vi "Patch data preview-Initialise all.vi"() -> (2 "VL array refs":T1[](array[typedef]), 3 "U8 Image ref":T1)   [LabVIEW 2020]
uses:
  <vilib>/vision/Image Controls.llb/IMAQ Image.ctl
  User Interface/Visualisation/Timelapse Viewer/Globals/gl_Time series viewer globals.vi
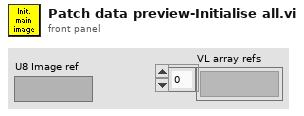
[diagram p1: front panel]
types:
  T1 = typedef "IMAQ Image.ctl" = refnum<image>
  T2 = typedef "Time series viewer refs.ctl" = cluster{"This VI":refnum<vi>, "Image control":refnum<vi>, "AVI Mode ind":refnum<vi>, "Play":refnum<vi>, "Stop":refnum<vi>, "Back":refnum<vi>, "Scrollbar":refnum<vi>, "Video length info":refnum<vi>, "Expected speed values":refnum<vi>, "Intensity":refnum<vi>, "Path":refnum<vi>, "Selection sliders":refnum<vi>, "Speed Graph ref":refnum<vi>, "Frame rate set (fps)":refnum<vi>, "Number of rows to generate":refnum<vi>, "VL Image Array":refnum<vi>, "Image Scrollbar":refnum<vi>, "Channel to load":refnum<vi>, "Colour":refnum<vi>}
  T3 = typedef "Channel to load.ctl" = enum16{"Show red channel", "Show green channel", "Show both channels"}
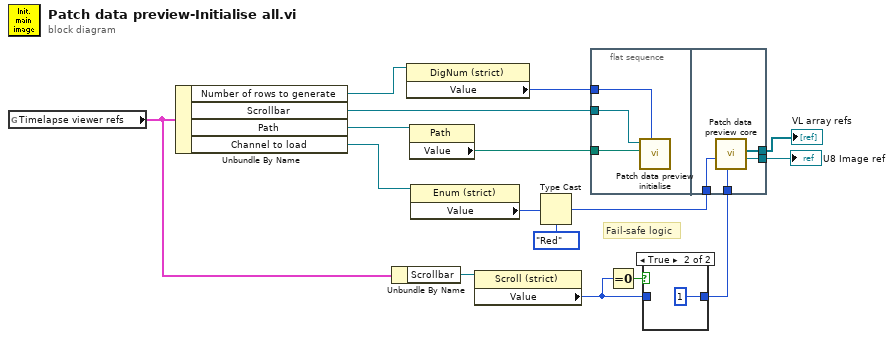
[diagram p0: block diagram]
diagram:
  # "Fail-safe logic"
  n1 = global read "gl_Time series viewer globals.vi" "Timelapse viewer refs"() -> (w5:T2)
  n2 = Unbundle By Name(w5) -> ("Number of rows to generate"=w12:refnum<vi>, "Scrollbar"=w9:refnum<vi>, "Path"=w10:refnum<vi>, "Channel to load"=w14:refnum<vi>)
  n3 = Unbundle By Name(w5) -> ("Scrollbar"=w8:refnum<vi>)
  n4 = property class="DigNum (strict)"(reference=w12) -> ("Value"=w13:i32)  [unwired: 1 in, 2 out]
  n5 = property class="Path"(reference=w10) -> ("Value"=w11:path)  [unwired: 1 in, 2 out]
  n6 = property class="Enum (strict)"(reference=w14) -> ("Value"=w15:T3)  [unwired: 1 in, 2 out]
  n7 = property class="Scroll (strict)"(reference=w8) -> ("Value"=w3:i32)  [unwired: 1 in, 2 out]
  n8 = Type Cast(type=enum16{"Red", "Green"}."Red" ("Channel to load"), x=w15) -> (*(type *) &x=w7:enum16{"Red", "Green"})
  n9 = flat-sequence {
    tunnel: w13 -> [w19]
    tunnel: w11 -> [w18]
    tunnel: w9 -> [w17]
    tunnel: w7 -> [w23]
    tunnel: w2 -> [w22]
    tunnel: [w21] -> w6
    tunnel: [w20] -> w1
    frame #0 {
      n10 = call "Patch data preview initialise.vi"("Number of rows to generate"=w19, "Dataset path"=w18, "Scrollbar ref"=w17) -> ()  [unwired: 8 in, 1 out]
    }
    frame #1 {
      n11 = call "Patch data preview core.vi"("Global cycle number among all trials"=w22, "Channel to load"=w23) -> ("Image ref (montage)"=w21:T1, "Array"=w20:T1[])  [unwired: 7 in, 1 out]
    }
  }
  n12 = Equal To 0?(x=w3) -> (x = 0?=w4:bool)
  n13 = case shown="True" w4 {
    tunnel: [w24 1 ("Value")] -> w2
    tunnel: w3 -> [w24 _]
    frame False {
    }
    frame True {
    }
  }
  "U8 Image ref" <- w6
  "VL array refs" <- w1
